vi "Motors FGV.vi"(6 "Action":T1, 8 "error in (no error)":errorcluster, 11 "Motor control in":T2) -> (0 "error out":errorcluster, 3 "Motor control out":T2)   [LabVIEW 2020]
uses:
  NI_DAQ/Libraries/NI DAQ/Controls/Motor controls---typedef.ctl
  controls/Motor FGV states ---typedef.ctl
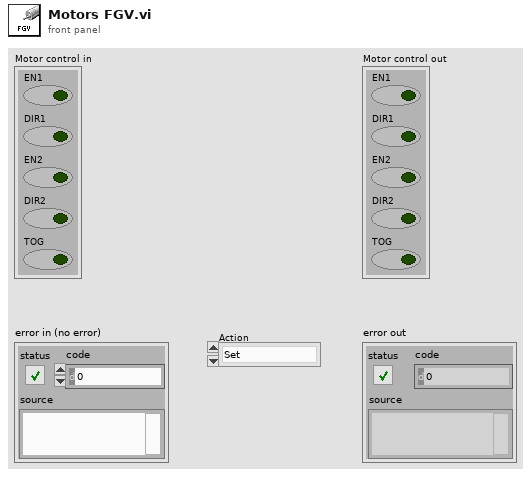
[diagram p1: front panel]
types:
  T1 = typedef "Motor FGV states ---typedef.ctl" = enum16{"Set", "Reset", "Get"}
  T2 = typedef "Motor controls---typedef.ctl" = cluster{"EN1":bool, "DIR1":bool, "EN2":bool, "DIR2":bool, "TOG":bool}
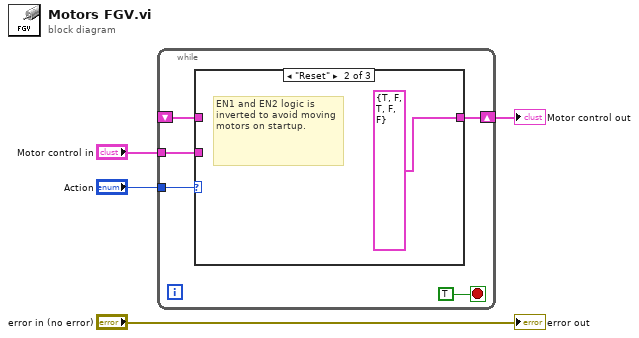
[diagram p0: block diagram]
diagram:
  n1 = while {
    tunnel: "Action" -> [w8]
    shift-right: [w7] -> w2
    shift-left: _ -> [w6]
    tunnel: "Motor control in" -> [w5]
    stop <- TRUE stop-if-true
    n2 = case shown="\"Reset\"" w8 {
      tunnel: [w10 T2 {"EN1"=TRUE, "DIR1"=FALSE, "EN2"=TRUE, "DIR2"=FALSE, "TOG"=FALSE} ("Motor control") w12] -> w7
      tunnel: w6 -> [_ _ w12]
      tunnel: w5 -> [w10 _ _]
      frame "Set", Default {
      }
      frame "Reset" {
        # "EN1 and EN2 logic is inverted to avoid moving motors on startup."
      }
      frame "Get" {
      }
    }
  }
  "Motor control out" <- w2
  "error out" <- "error in (no error)"
